vi "save ini configuration to image file path.vi"(11 "exclusion regexp array":string[](array[string])) -> ()   [LabVIEW 2012]
doc: "SciScan 1.0 151216"
uses:
  GFG/GFGpathGet.vi
  GFG/GFG library.lvlib
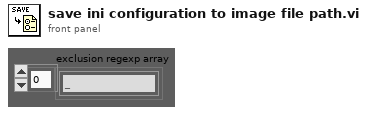
[diagram p1: front panel]
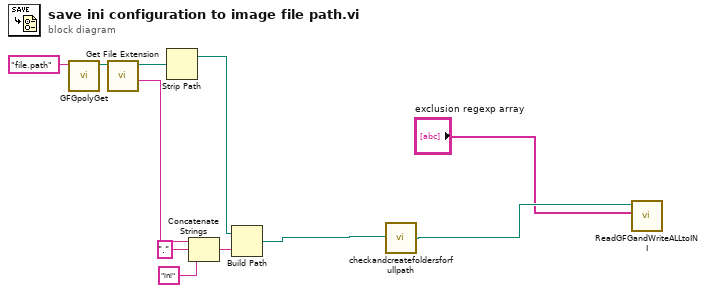
[diagram p0: block diagram]
diagram:
  n1 = call-poly "GFGpolyGet.vi"("Variable Name in"="file.path") -> ("Path"=w7:path)  [unwired: 8 in, 2 out]
  n2 = call <vilib>:"Get File Extension.vi"("file"=w7) -> ("filename without extension"=w8:string)  [unwired: 7 in, 3 out]
  n3 = Strip Path(path=w7) -> (stripped path=w9:path)  [unwired: 1 out]
  n4 = Concatenate Strings(w8, "." ("string"), "ini" ("string")) -> (w10:string)
  n5 = Build Path(base path=w9, name or relative path=w10) -> (appended path=w3:path)
  n6 = call "checkandcreatefoldersforfullpath.vi"("Path IN"=w3) -> ("Path OUT"=w2:path)  [unwired: 4 in]
  n7 = call "ReadGFGandWriteALLtoINI.vi"("exclusion regexp array"="exclusion regexp array", "Path"=w2) -> ()  [unwired: 9 in, 1 out]
